vi "Reshape mov cor data.vi"(9 "Logging queue element in":T1={"Imaging Protocol"=enum."Live Imaging", "Number of Trials"=0, "Frame Size"=512, "# Averaged frames"=0, "Dwell time (us)"=0.0, "Index of Z-plane"=0, "Timelapse?"=FALSE, "Logging process is active"=FALSE, "Speed logging enabled"=FALSE, "tdms file ref"=refnum, "path"=path "", "Trial Number"=0, "Expected # points acquired"=FALSE, "Manually stopped"=FALSE, "Ch0 data"=[], "Ch1 data"=[], "Ref Data"=[], "Last trial"=FALSE, "Ref Dwell time (us)"=0.0, "# Ref Averaged frames"=0, "Ref X Length"=0, "Ref Y Length"=0, "Points acquired"={"Ch0 last trial"=0, "Ch1 last trial"=0, "All trials"=0}} {"Ref Dwell time (us)" format="%#.6g"; "Frame Size" items=["100X100"=100, "128X128"=128, "200X200"=200, "256X256"=256, "512X512"=512, "1024x1024"=1024, "2048x2048"=2048]; "Dwell time (us)" format="%#.6g"}, 11 "Data":T5) -> (0 "Ch1- Green Ref":i16[][](array[numeric]), 1 "Ch0-Red Ref":i16[][](array[numeric]))   [LabVIEW 2017]
uses:
  Typedefs/Frame data dual cluster.ctl
  Typedefs/Logging queue element.ctl
  Typedefs/Imaging Protocols enum.ctl
  Typedefs/Frame Size.ctl
  Typedefs/Acquired points count.ctl
panel:
  # "SUBROUTINE VI"
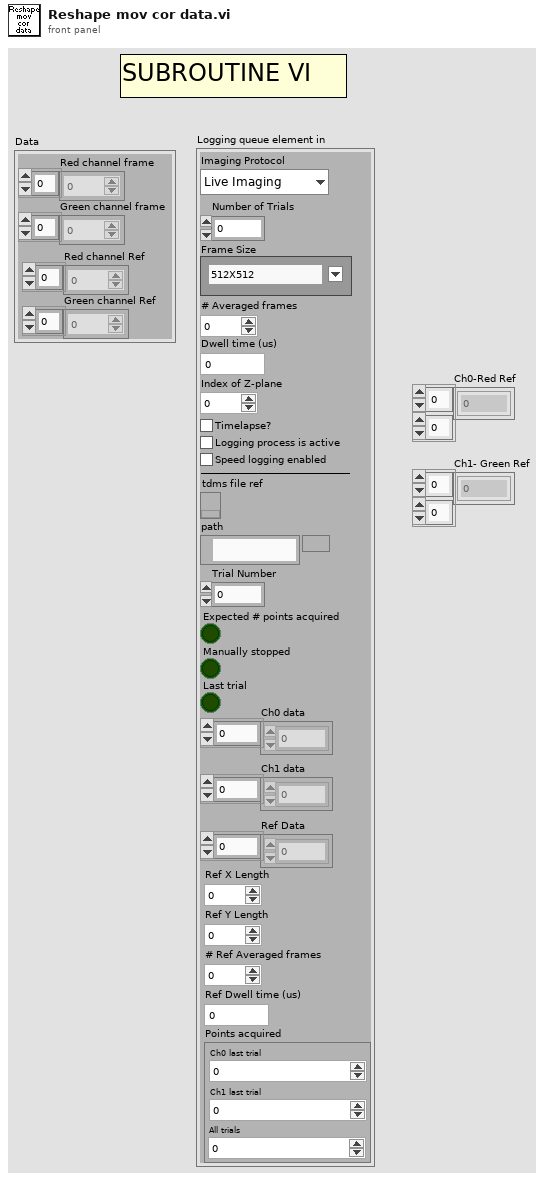
[diagram p1: front panel]
types:
  T1 = typedef "Logging queue element.ctl" = cluster{"Imaging Protocol":T2, "Number of Trials":u16, "Frame Size":T3, "# Averaged frames":u16, "Dwell time (us)":dbl, "Index of Z-plane":i32, "Timelapse?":bool, "Logging process is active":bool, "Speed logging enabled":bool, "tdms file ref":refnum<k34>, "path":path, "Trial Number":i32, "Expected # points acquired":bool, "Manually stopped":bool, "Ch0 data":u32[], "Ch1 data":u32[], "Ref Data":u32[], "Last trial":bool, "Ref Dwell time (us)":dbl, "# Ref Averaged frames":u16, "Ref X Length":u16, "Ref Y Length":u16, "Points acquired":T4}
  T2 = typedef "Imaging Protocols enum.ctl" = enum16{"AOL Z-Stack", "Motor Z Stack", "Functional Acquisition", "Single Plane Acquisition", "Volume Acquisition", "Live Imaging", "Live Plane Imaging", "Live Volume Imaging"}
  T3 = typedef "Frame Size.ctl" = u16
  T4 = typedef "Acquired points count.ctl" = cluster{"Ch0 last trial":u64, "Ch1 last trial":u64, "All trials":u64}
  T5 = typedef "Frame data dual cluster.ctl" = cluster{"Red channel frame":dbl[], "Green channel frame":dbl[], "Red channel Ref":dbl[], "Green channel Ref":dbl[]}
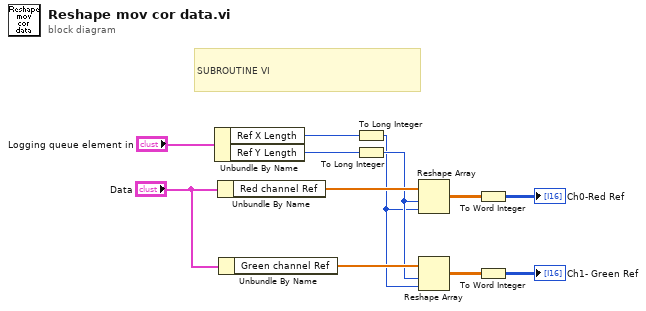
[diagram p0: block diagram]
diagram:
  # "SUBROUTINE VI"
  n1 = Unbundle By Name("Logging queue element in") -> ("Ref X Length"=w6:u16, "Ref Y Length"=w5:u16)
  n2 = Unbundle By Name("Data") -> ("Red channel Ref"=w10:dbl[])
  n3 = Unbundle By Name("Data") -> ("Green channel Ref"=w9:dbl[])
  n4 = To Long Integer(number=w6) -> (32bit integer=w3:i32)
  n5 = To Long Integer(number=w5) -> (32bit integer=w4:i32)
  n6 = Reshape Array(w10, w4, w3) -> (w12:dbl[][])
  n7 = Reshape Array(w9, w4, w3) -> (w11:dbl[][])
  n8 = To Word Integer(number=w12) -> (16bit integer=→"Ch0-Red Ref":i16[][])
  n9 = To Word Integer(number=w11) -> (16bit integer=→"Ch1- Green Ref":i16[][])
